vi "testDataPass_v3,0_rt.vi"() -> ()   [LabVIEW 2014]
panel:
  out "error out 2":errorcluster
  in  "stop":bool
  out "error out":errorcluster
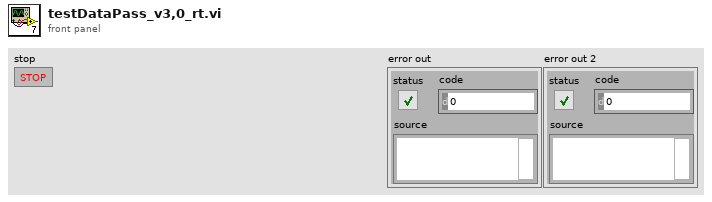
[diagram p1: front panel]
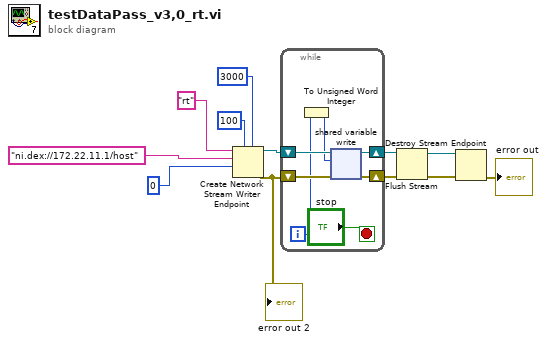
[diagram p0: block diagram]
diagram:
  n1 = Create Network Stream Writer Endpoint(5:3000 ("timeout in ms (-1)"), 7:100 ("writer buffer size"), 9:u16 0, 10:"ni.dex://172.22.11.1/host" ("reader url"), 11:"rt" ("writer name")) -> (0:w9:errorcluster, 3:w10:refnum<k21>)  [unwired: 2 in]
  "error out 2" <- w9
  n2 = while {
    shift-right: [w16] -> w7
    shift-left: w10 -> [w19]
    shift-right: [w15] -> w6
    shift-left: w9 -> [w18]
    i -> [w14]
    stop <- "stop" stop-if-true
    n3 = To Unsigned Word Integer(number=w14) -> (unsigned 16bit integer=w17:u16)
    n4 = shared-variable-write(w19, w18, w17) -> (w16:refnum<k21>, w15:errorcluster)  [unwired: 1 in, 1 out]
  }
  n5 = Flush Stream(8:w6, 11:w7) -> (0:w5:errorcluster, 3:w4:refnum<k21>)  [unwired: 2 in, 1 out]
  n6 = Destroy Stream Endpoint(8:w5, 11:w4) -> (0:→"error out":errorcluster)
